vi "Generate Test Channel Values (SubVI).vi"(1 "Aliases in":string[](array[string])) -> (0 "Test Channel Values out":dbl[](array[numeric]))   [LabVIEW 2019, in "FPGA Addon Test Class.lvclass"]
uses:
  FPGA Addon Test Class.lvclass
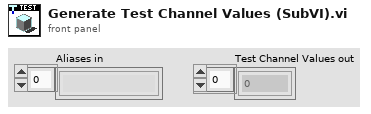
[diagram p1: front panel]
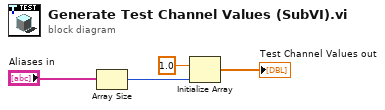
[diagram p0: block diagram]
diagram:
  n1 = Array Size(array="Aliases in") -> (size(s)=w3:i32)
  n2 = Initialize Array(1.0 ("Value"), w3) -> (→"Test Channel Values out":dbl[])
